vi "LTESaveDataImg1.vi"(7 "Boolean":bool, 8 "error in":errorcluster, 9 "varName":string, 10 "real1":cdb[](array[numeric])=[1.0+0.0i, 2.0+0.0i, 3.0+0.0i], 11 "Path":path=path "C:/Users/Administrator/Desktop") -> (0 "error IO":errorcluster)   [LabVIEW 2015]
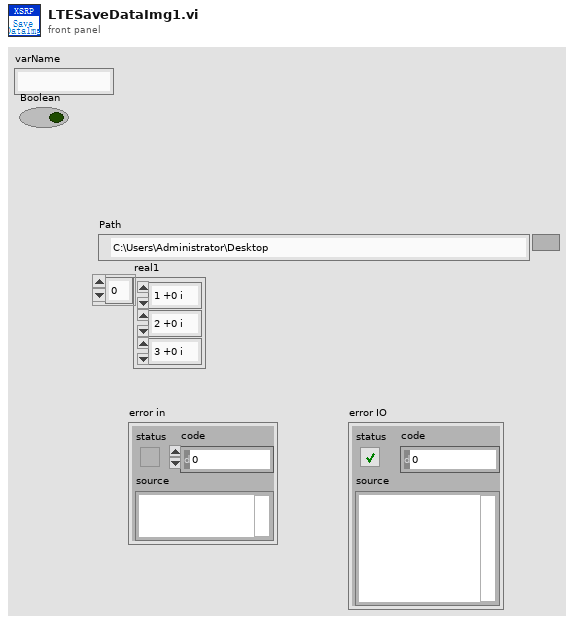
[diagram p1: front panel]
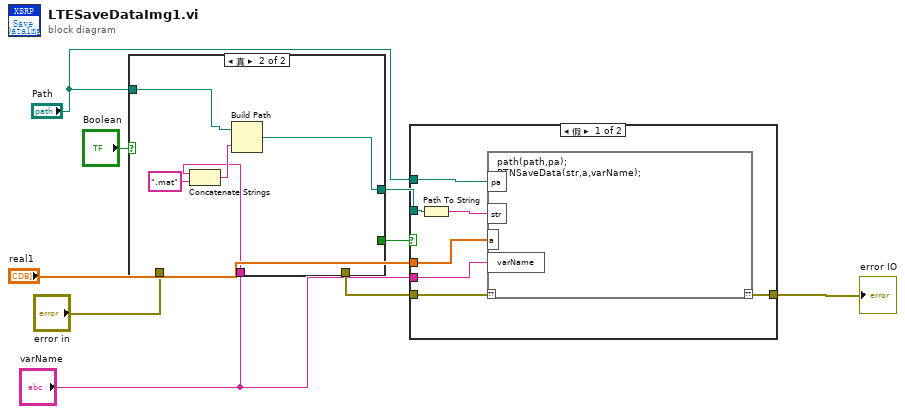
[diagram p0: block diagram]
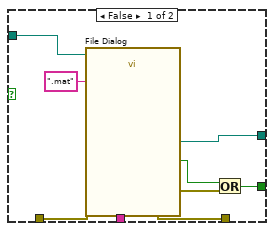
[diagram p2: hidden frame]
diagram:
  n1 = case shown="真" "Boolean" {
    tunnel: [w16 w18] -> w9
    tunnel: [w14 _] -> w8
    tunnel: "Path" -> [w13 w19]
    tunnel: "error in" -> [w12 _]
    tunnel: [w11 _] -> w3
    tunnel: "varName" -> [_ w17]
    frame False {
      n2 = call "File Dialog"("start path"=w13, "error in"=w12, "pattern (all files)"=".mat") -> ("selected path"=w16:path, "cancelled"=w10:bool, "error out"=w11:errorcluster)  [unwired: 9 in, 1 out]
      n3 = Or(x=w10, y=w11) -> (x .or. y?=w14:bool)
    }
    frame True {
      n4 = Concatenate Strings(w17, ".mat" ("string")) -> (w20:string)
      n5 = Build Path(base path=w19, name or relative path=w20) -> (appended path=w18:path)
    }
  }
  n6 = case shown="假" w8 {
    tunnel: w9 -> [w28 _]
    tunnel: "Path" -> [w26 _]
    tunnel: "real1" -> [w25 _]
    tunnel: w3 -> [w24 w29]
    tunnel: [w23 w29] -> w5
    tunnel: "varName" -> [w22 _]
    frame False {
      n7 = Path To String(path=w28) -> (string=w27:string)
      n8 = script code="path(path,pa);\nBTNSaveData(str,a,varName);"("??"=w24, "pa"=w26, "a"=w25, "str"=w27, "varName"=w22) -> ("??"=w23:errorcluster)
    }
    frame True {
    }
  }
  "error IO" <- w5
